vi "LV SCISDK Get Parameter Integer.vi"(8 "error in (no error)":errorcluster, 10 "handle":u64, 11 "Path":string) -> (0 "error out":errorcluster, 1 "function return":i32, 2 "handle out":u64, 3 "value":i32)   [LabVIEW 2021, in "SciSDK_Labview.lvlib"]
doc: "SCISDKLABVIEW_DLL_API int LV_SCISDK_GetParameterInteger(char* Path, int* value, void* handle);"
uses:
  SciSDK_Labview.lvlib
  <userlib>/SciSDK_Labview/SciSDK_Labview.dll
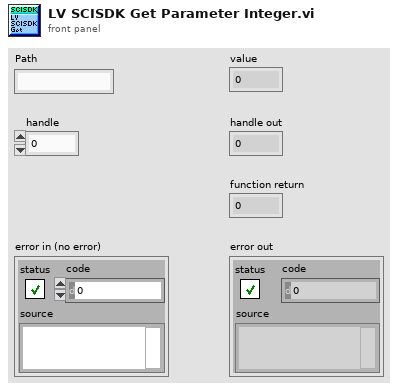
[diagram p1: front panel]
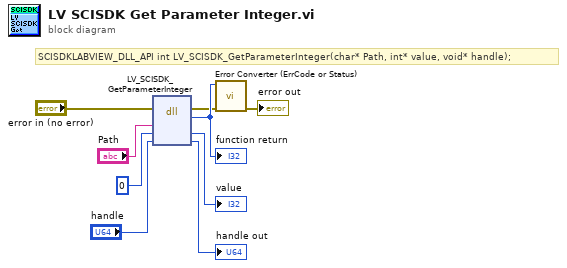
[diagram p0: block diagram]
diagram:
  # "SCISDKLABVIEW_DLL_API int LV_SCISDK_GetParameterInteger(char* Path, int* value, void* handle);"
  n1 = dll-call lib="C:/Program Files/National Instruments/LabVIEW 2021/user.lib/SciSDK_Labview/SciSDK_Labview.*" fn="LV_SCISDK_GetParameterInteger"(error in="error in (no error)", "Path"="Path", "value"=0, "handle"="handle") -> (error out=w2:errorcluster, w9:i32, "value"=→"value":i32, "handle"=→"handle out":u64)  [unwired: 3 in, 1 out]
  "function return" <- w9
  n2 = call <userlib>:"Error Converter (ErrCode or Status).vi"("error in (no error)"=w2, "error code"=w9) -> ("error out"=→"error out":errorcluster)  [unwired: 9 in]
